vi "Robot Main.vi"   [LabVIEW 2013]
doc: "This VI imlements the framework and scheduler for your robotics program. It should not be necessary to modify the framework. You are expected to add your code to the VIs called from Robot Main, the ones located in the Team Code within the project."
panel:
  # "2014 Über Code"
  # "Version 0.7_Sat: 2-8-14"
  # "Todo"
  # "Controls"
  # "PWM"
  # "DIO"
  # "Relay"
  # "Analog"
  # "Solenoid"
  # "- Clean Up Code\n- Empty old code out\n- Prepare Vision\n- Implement new systems with joystick buttons/axis\n-Make loops communicate to eachother\n-Add working auto distance for shooting\n-Finish (un-tuned) code\n-Dashboard comms\n-Custom Dashboard Project\n-use hat switch?"
  # "Joystick 1\nX Axis: Arcade Drive \nY Axis: Arcade Drive \nZ Axis:\nButton 1: Hold Position Toggle\nButton 2:\nButton 3:\nButton 4:\nButton 5:\nButton 6: \nButton 7: Shift High\nButton 8: Toggle Vision\nButton 9: Go To Shoot Location\nButton 10: \nButton 11: Disable Vision & GoTo DC\nButton 12: Shift Low"
  # "Joystick 2\nX Axis: \nY Axis: Belts Manual Override/DC \nZ Axis: Tune Belt Speed\nButton 1: \nButton 2: \nButton 3: \nButton 4: \nButton 5: Belts Driver Control\nButton 6: Belts Manual Override\nButton 7: \nButton 8: \nButton 9: \nButton 10: \nButton 11: Pickup (For Passing)\nButton 12: Pass"
  # "Joystick 3\nX Axis: \nY Axis: Pickup Arm Manual Overide\nZ Axis: Tune Pickup Arm Pickup Height\nButton 1: Shoot\nButton 2: Load\nButton 3: \nButton 4: \nButton 5: Arm Driver Control\nButton 6: Arm Manual Override\nButton 7: \nButton 8: \nButton 9: Home Arm\nButton 10: \nButton 11: \nButton 12:"
  # "1 a): Right Front Drive\n1 b): Right Rear Drive\n2 a): Left Front Drive\n2 b): Left Rear Drive\n3 a): Right Pickup Motor\n3 b): Left Pickup Motor\n     4: Pickup Belt\n     5:  \n     6: \n     7: \n     8: \n     9: \n   10:"
  # "1: Right Drive Encoder A\n  2: Right Drive Encoder B\n  3: Left Drive Encoder A  \n  4: Left Drive Encoder B\n  5: Pickup Motor Encoder A\n  6: Pickup Motor Encoder B\n  7: Shooter Magnetic Sensor R-Up\n  8: Shooter Magnetic Sensor R-Down\n  9: Shooter Magnetic Sensor L-Up\n10: Shooter Magnetic Sensor L-Down\n11: Lock Magnetic Sensor (extended)\n12: Holding Light Sensor\n13: \n14: Pneumatic Pressure Switch"
  # "1: Compressor Spike\n2:\n3:\n4:\n5:\n6:\n7:\n8:"
  # "1:\n2:\n3:\n4:\n5:\n6:\n7:\n8:"
  # "1: Shifter A\n2: Shifter B\n3: Shooter A\n4: Shooter B\n5: Lock A\n6: Lock B\n7:\n8:"
  # "Revision History"
  # "0.1\n-Blank(ish) structure\n0.2\n-Cleaned out old game-specific code\n-Updated VIs\n-Added vision/changed vision\n-finished distance\n0.3\n-modified teleop and structure\n-basic teleop complete, auto ready for setup\n-goto shoot vi added\n-configured begin vi\n-worked on structure/arm vi\n0.4\n-edited goto shoot vi\n-revised vision calculating vi\n-changed joystick layouts"
  # "-no longer use holding sensor\n-arm code done (untuned)\n-belt code done (untuned)\n-shooter code done (untuned)\n-go to shoot code done (untuned)\n-vision done (untuned)\n-constants needing tuning changed to controls\n-made goto shoot change to hold position when done\n0.5\n-removed 3 of the 4 piston sensors :'(\n-shooter piston code compensates for ^\n-edited build custom dashboard data vi\n-updated arm saftey to match dashboard\n0.6\n-Misc. improvements"
  # "0.7\n-Added more magnetic piston sensors :)\n-Edited code to compensate for ^\n-changed axis 3 to 4 because of new joysticks\n-fixed bug in belt code\n-changed pickup arm hold position code\n-removed unnecessary support code VIs\n-added lock engaged sensor\n-changed joystick 1 layout\n-updated begin and finish VIs\n-lock leaves shoot after shoots\n-updated shoot safely.vi\n-incorporated error filters on axes"
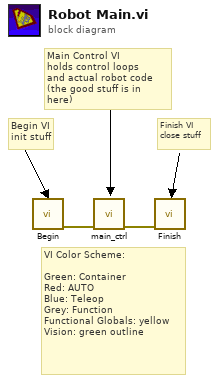
[diagram p0: block diagram]
diagram:
  # "Finish VI\nclose stuff"
  # "Main Control VI\nholds control loops\nand actual robot code\n(the good stuff is in here)"
  # "Begin VI\ninit stuff"
  # "VI Color Scheme:\n\nGreen: Container\nRed: AUTO\nBlue: Teleop\nGrey: Function\nFunctional Globals: yellow\nVision: green outline"
  n1 = call "Begin.vi"() -> ("error out"=w2:errorcluster)  [unwired: 1 in, 10 out]
  n2 = call "main_ctrl.vi"("error in"=w2) -> ("error out"=w1:errorcluster)  [unwired: 10 in]
  n3 = call "Finish.vi"("error in"=w1) -> ()  [unwired: 7 in]
